vi "ChemProj.vi"() -> ()   [LabVIEW 2012]
uses:
  <userlib>/ImageProcessing/InitCamera_NTSC.vi
  <userlib>/ImageProcessing/FilterGreenPlane.vi
  <userlib>/ImageProcessing/FilterRedPlane.vi
panel:
  out "Question":string
  out "Element Found":string[](array[string])
  out "Grade":dbl
  out "Element":string[](array[string])
  out "indexsWhereTrue":i32[](array[numeric])
  out "Min":dbl[](array[numeric])
  out "Max":dbl[](array[numeric])
  out "x+y":dbl[](array[numeric])
  out "S4":dbl[](array[numeric])
  out "S3":dbl[](array[numeric])
  out "S2":dbl[](array[numeric])
  out "S1":dbl[](array[numeric])
  in  "Path":path
  out "Periodic":string[][](array[string])
  out "image 2":picture
  out "Ra4":dbl
  out "Ra3":dbl
  out "Ra2":dbl
  out "Ra1":dbl
  out "A4":dbl
  out "A3":dbl
  out "A2":dbl
  out "A1":dbl
  out "a4":dbl
  out "a3":dbl
  out "a2":dbl
  out "a1":dbl
  out "Centroid 4":cluster{"X":dbl, "Y":dbl}
  out "Centroid 3":cluster{"X":dbl, "Y":dbl}
  out "Centroid 2":cluster{"X":dbl, "Y":dbl}
  out "Centroid":cluster{"X":dbl, "Y":dbl}
  out "initialized array 2":dbl[][](array[numeric])
  out "image":picture
  in  "Stop":bool
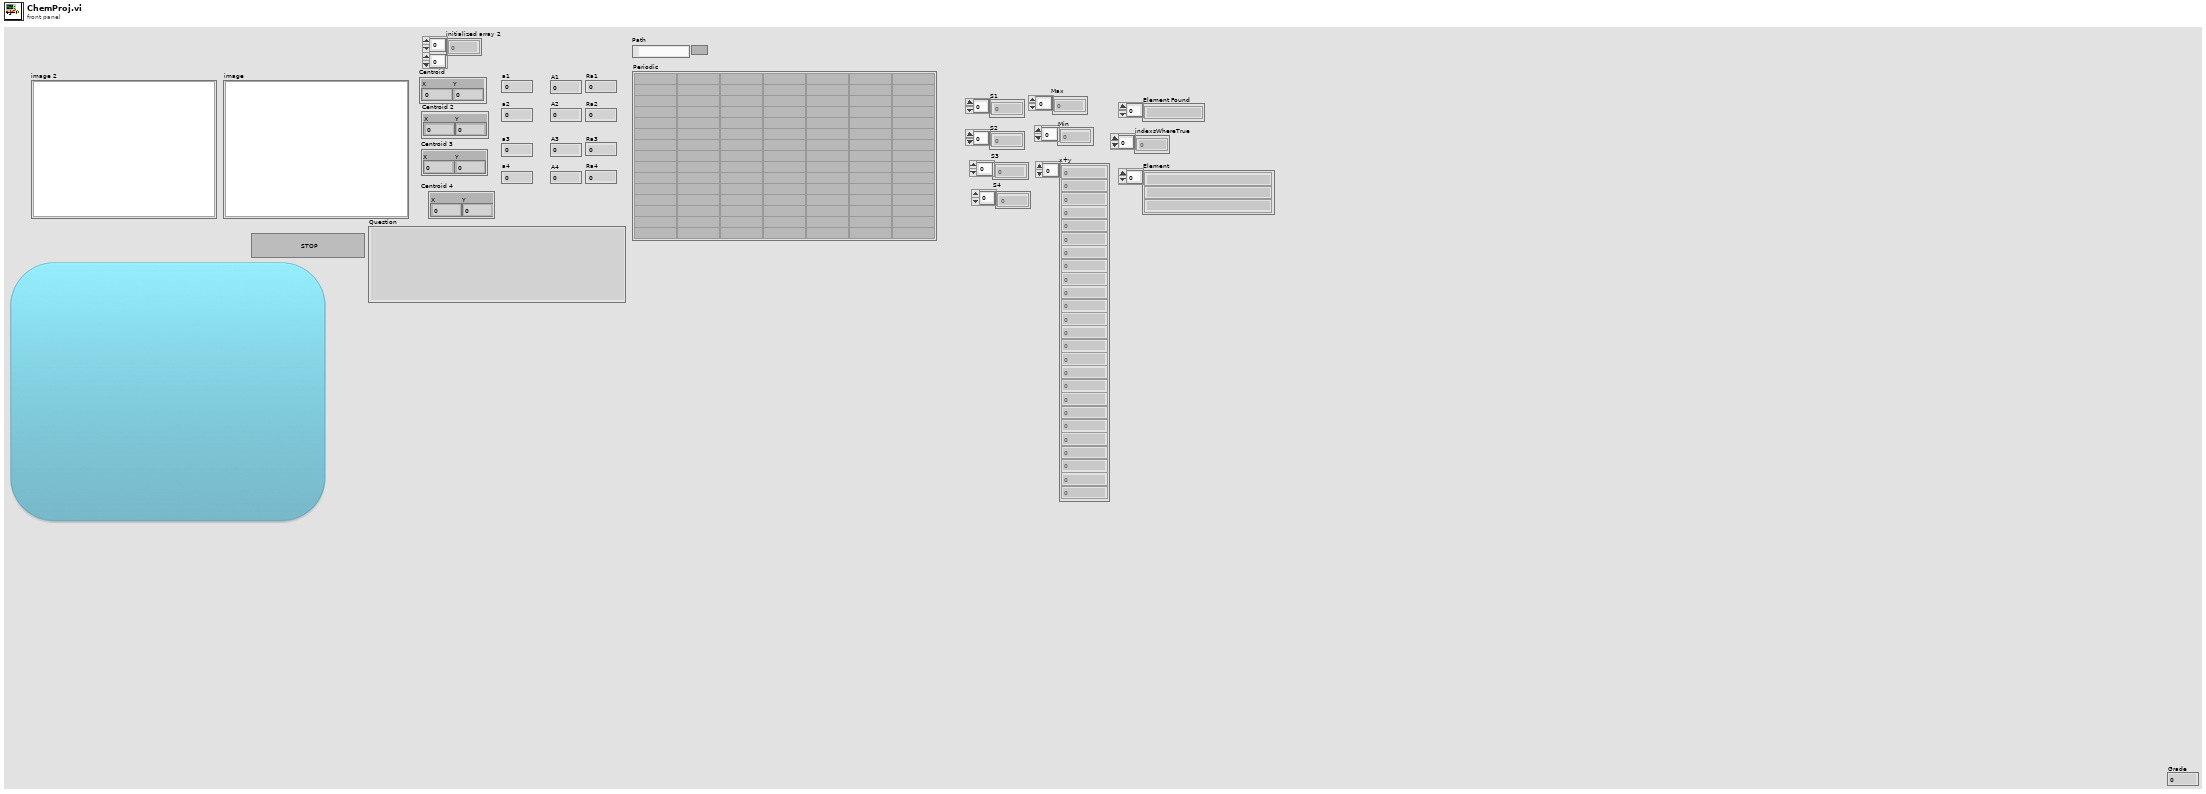
[diagram p1: front panel]
types:
  T1 = typedef "QT_Ref.ctl" = refnum<k1>
  T2 = cluster{"Width":u16, "Style":enum32{"Solid", "Dash", "Dot", "DashDot", "DashDotDot"}}
  T3 = typedef "QT_Image.ctl" = cluster{"Width":i32, "Height":i32, "Depth":i32, "data":u8[], "Compressed data":u8[], "Color table":u32[], "Duration":i32, "Options":i32, "Timestamp":i32, "ID":i32, "Reserved":i32, "Dialogs":u32}
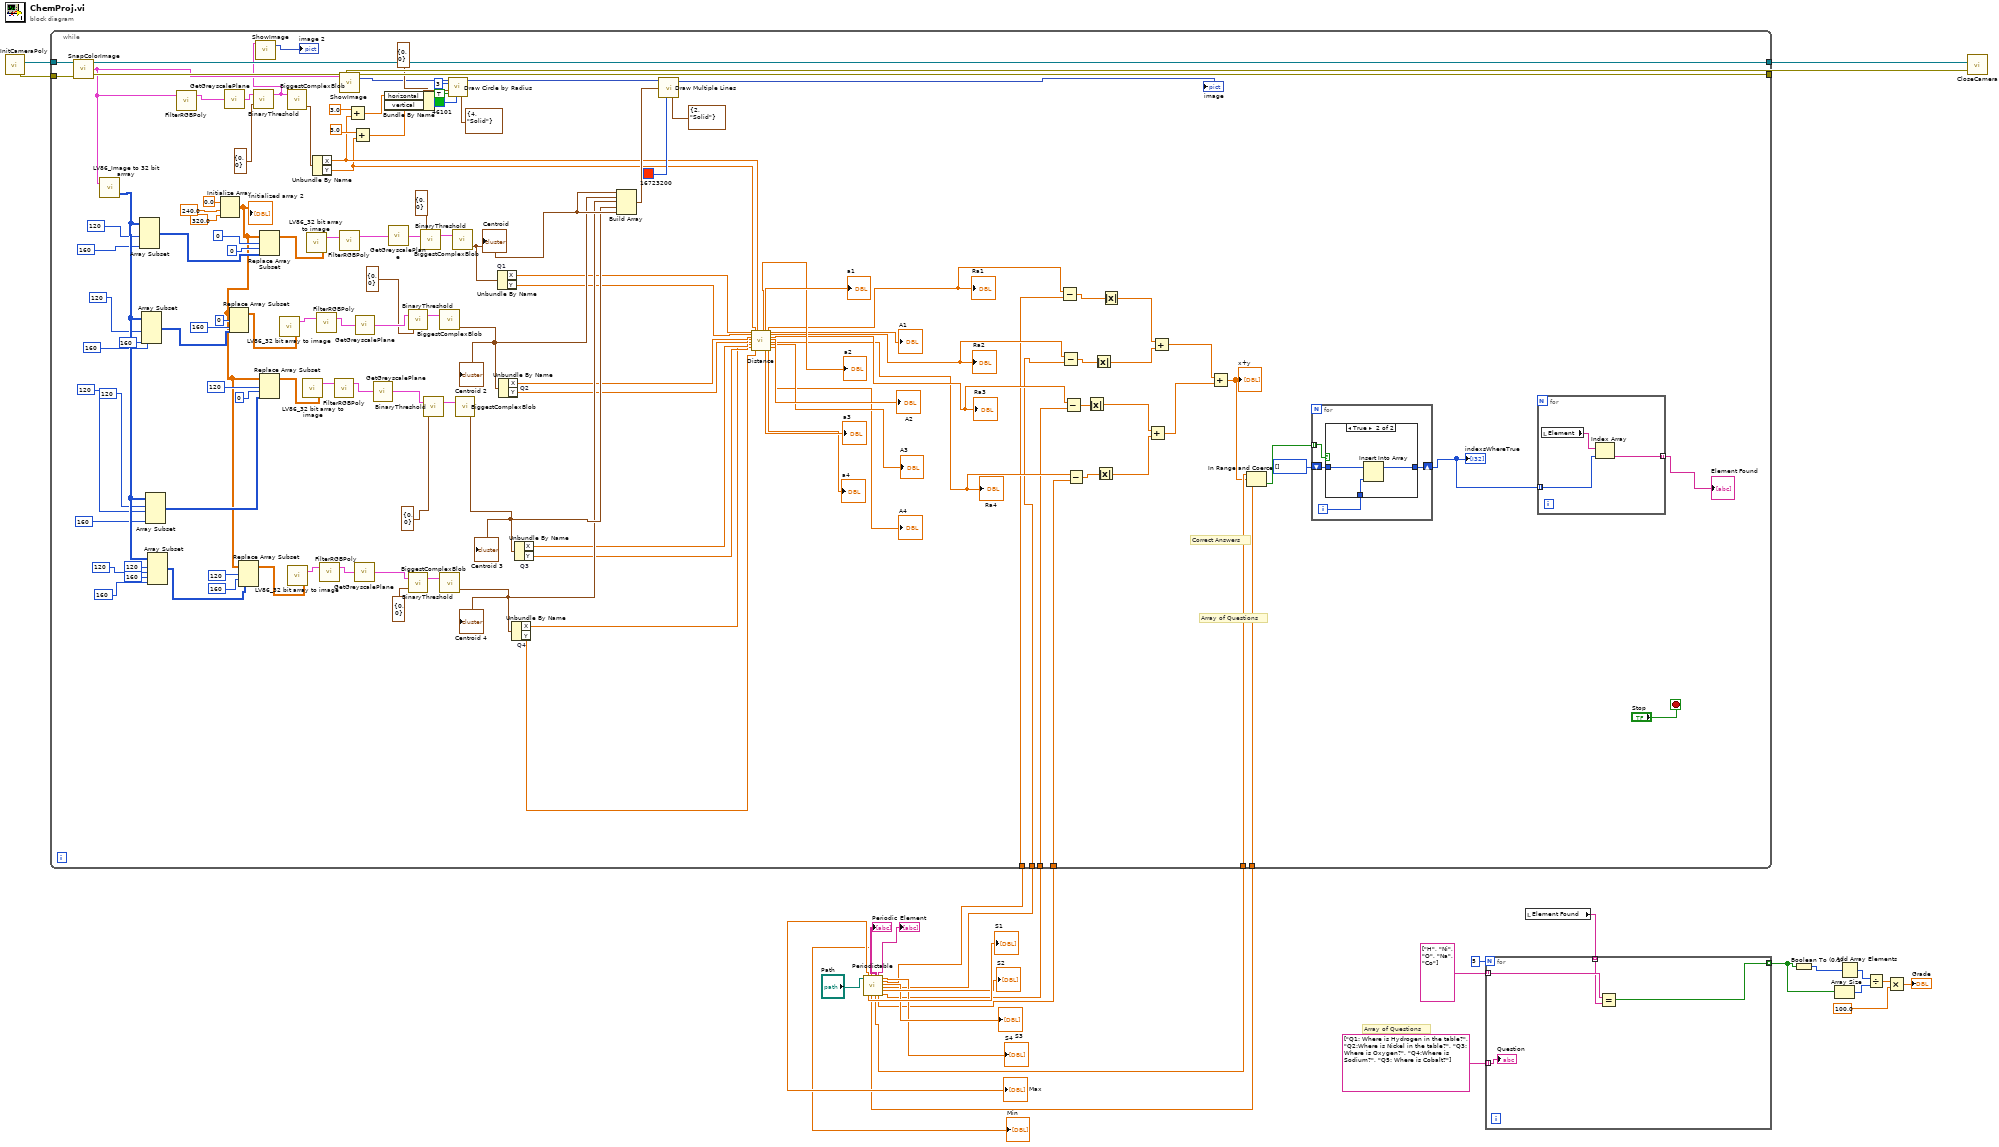
[diagram p0: block diagram]
diagram:
  # "Array of Questions"
  n1 = call-poly <userlib>:"InitCameraPoly.vi"() -> ("error out"=w27:errorcluster, "QT Ref Out"=w28:T1)  [unwired: 2 in]
  n2 = call "Periodictable.vi"("Path"="Path") -> ("Max"=→"Max":dbl[], "S1"=→"S1":dbl[], "Min"=→"Min":dbl[], "Array"=w17:dbl[], "Periodic"=→"Periodic":string[][], "Array 2"=w16:dbl[], "Element"=→"Element":string[], "Array 3"=w12:dbl[], "S4"=→"S4":dbl[], "Array 6"=w15:dbl[], "S3"=→"S3":dbl[], "Array 5"=w14:dbl[], "S2"=→"S2":dbl[], "Array 4"=w13:dbl[])  [unwired: 5 in]
  n3 = while {
    tunnel: w27 -> [w158]
    tunnel: w28 -> [w157]
    tunnel: [w156] -> w29
    tunnel: [w155] -> w30
    tunnel: w15 -> [w51]
    tunnel: w14 -> [w50]
    tunnel: w13 -> [w49]
    tunnel: w12 -> [w48]
    tunnel: w16 -> [w37]
    tunnel: w17 -> [w36]
    stop <- "Stop" stop-if-true
    # "Correct Answers"
    # "Array of Questions"
    n4 = call <userlib>:"SnapColorImage.vi"("error in (no error)"=w158, "QT Ref In"=w157) -> ("error out"=w156:errorcluster, "Image Out"=w89:T3, "QT Ref Out"=w155:T1)  [unwired: 1 in]
    n5 = call <userlib>:"LV86_Image to 32 bit arrray.vi"("Image In"=w89) -> ("Intensity Graph"=w153:u32[][])  [unwired: 1 in, 1 out]
    n6 = Array Subset(array=w153, length (row)=120 ("length"), length (col)=160 ("length")) -> (w129:u32[][])  [unwired: 2 in]
    n7 = Array Subset(array=w153, length (row)=120 ("length"), index (col)=160 ("index"), length (col)=160 ("length")) -> (w140:u32[][])  [unwired: 1 in]
    n8 = Array Subset(array=w153, index (row)=120 ("index"), length (row)=120 ("length"), length (col)=160 ("length")) -> (w123:u32[][])  [unwired: 1 in]
    n9 = Array Subset(array=w153, index (row)=120 ("index"), length (row)=120 ("length"), index (col)=160 ("index"), length (col)=160 ("length")) -> (w120:u32[][])
    n10 = call-poly <userlib>:"FilterRGBPoly.vi"("Image in"=w89) -> ("Image out"=w92:T3)  [unwired: 1 in, 1 out]
    n11 = Initialize Array(0.0 ("element"), 240.0 ("element"), 320.0 ("element")) -> (w119:dbl[][])
    "initialized array 2" <- w119
    n12 = call <userlib>:"GetGreyscalePlane.vi"("Image In"=w92) -> ("Greyscale  Out"=w76:T3)
    n13 = Replace Array Subset(array=w119, new element=w140, index (row)=0, index (col)=160 ("index (row)")) -> (w139:dbl[][])
    n14 = Replace Array Subset(array=w119, new element=w120, index (row)=120, index (col)=160 ("index (row)")) -> (w117:dbl[][])
    n15 = call <userlib>:"BinaryThreshold.vi"("threshold"=cluster{u8, u8} {0, 0}, "Image In"=w76) -> ("Image Out"=w74:T3)  [unwired: 1 in]
    n16 = call <userlib>:"ShowImage.vi"("Image"=w74) -> ("image"=→"image 2":picture)  [unwired: 2 in, 1 out]
    n17 = Replace Array Subset(array=w119, new element=w129, index (row)=0, index (col)=0 ("index (row)")) -> (w128:dbl[][])
    n18 = Replace Array Subset(array=w119, new element=w123, index (row)=120, index (col)=0 ("index (row)")) -> (w118:dbl[][])
    n19 = call <userlib>:"LV86_32 bit array to image.vi"("Intensity Graph"=w139) -> ("Image Out"=w116:T3)  [unwired: 2 in]
    n20 = call <userlib>:"BiggestComplexBlob.vi"("Image in"=w74) -> ("Centroid"=w90:cluster{"X":dbl, "Y":dbl})  [unwired: 1 in, 2 out]
    n21 = call <userlib>:"LV86_32 bit array to image.vi"("Intensity Graph"=w117) -> ("Image Out"=w114:T3)  [unwired: 2 in]
    n22 = call <userlib>:"LV86_32 bit array to image.vi"("Intensity Graph"=w118) -> ("Image Out"=w115:T3)  [unwired: 2 in]
    n23 = call <userlib>:"LV86_32 bit array to image.vi"("Intensity Graph"=w128) -> ("Image Out"=w127:T3)  [unwired: 2 in]
    n24 = Unbundle By Name(w90) -> ("X"=w73:dbl, "Y"=w72:dbl)
    n25 = call-poly <userlib>:"FilterRGBPoly.vi"("Image in"=w116) -> ("Image out"=w113:T3)  [unwired: 1 in, 1 out]
    n26 = call-poly <userlib>:"FilterRGBPoly.vi"("Image in"=w114) -> ("Image out"=w111:T3)  [unwired: 1 in, 1 out]
    n27 = call-poly <userlib>:"FilterRGBPoly.vi"("Image in"=w115) -> ("Image out"=w112:T3)  [unwired: 1 in, 1 out]
    n28 = call <userlib>:"ShowImage.vi"("Image"=w89) -> ("image"=w77:picture)  [unwired: 2 in, 1 out]
    n29 = call-poly <userlib>:"FilterRGBPoly.vi"("Image in"=w127) -> ("Image out"=w126:T3)  [unwired: 1 in, 1 out]
    n30 = Add(x=3.0, y=w73) -> (x+y=w83:dbl)
    n31 = Add(x=3.0, y=w72) -> (x+y=w82:dbl)
    n32 = call <userlib>:"GetGreyscalePlane.vi"("Image In"=w111) -> ("Greyscale  Out"=w105:T3)
    n33 = call <userlib>:"GetGreyscalePlane.vi"("Image In"=w113) -> ("Greyscale  Out"=w107:T3)
    n34 = call <userlib>:"GetGreyscalePlane.vi"("Image In"=w112) -> ("Greyscale  Out"=w106:T3)
    n35 = Bundle By Name(cluster=cluster{"horizontal":i16, "vertical":i16} {"horizontal"=0, "vertical"=0} ("pixel center"), "horizontal"=w83, "vertical"=w82) -> (w87:cluster{"horizontal":i16, "vertical":i16})
    n36 = call <userlib>:"GetGreyscalePlane.vi"("Image In"=w126) -> ("Greyscale  Out"=w125:T3)
    n37 = call <userlib>:"BinaryThreshold.vi"("threshold"=cluster{u8, u8} {0, 0}, "Image In"=w107) -> ("Image Out"=w110:T3)  [unwired: 1 in]
    n38 = call <userlib>:"BinaryThreshold.vi"("threshold"=cluster{u8, u8} {0, 0}, "Image In"=w105) -> ("Image Out"=w108:T3)  [unwired: 1 in]
    n39 = call <userlib>:"BinaryThreshold.vi"("threshold"=cluster{u8, u8} {0, 0}, "Image In"=w125) -> ("Image Out"=w124:T3)  [unwired: 1 in]
    n40 = call <userlib>:"BinaryThreshold.vi"("threshold"=cluster{u8, u8} {0, 0}, "Image In"=w106) -> ("Image Out"=w109:T3)  [unwired: 1 in]
    n41 = call <userlib>:"BiggestComplexBlob.vi"("Image in"=w110) -> ("Centroid"=w95:cluster{"X":dbl, "Y":dbl})  [unwired: 1 in, 2 out]
    "Centroid 2" <- w95
    n42 = call <userlib>:"BiggestComplexBlob.vi"("Image in"=w108) -> ("Centroid"=w93:cluster{"X":dbl, "Y":dbl})  [unwired: 1 in, 2 out]
    "Centroid 4" <- w93
    n43 = call <vilib>:"Draw Circle by Radius.vi"("pen"=T2 {"Width"=4, "Style"=enum."Solid"}, "color(black)"=u32 46101, "fill?(F)"=TRUE, "pixel center"=w87, "radius"=i16 3, "picture"=w77) -> ("new picture"=w88:picture)  [unwired: 5 in]
    n44 = call <userlib>:"BiggestComplexBlob.vi"("Image in"=w124) -> ("Centroid"=w96:cluster{"X":dbl, "Y":dbl})  [unwired: 1 in, 2 out]
    "Centroid" <- w96
    n45 = call <userlib>:"BiggestComplexBlob.vi"("Image in"=w109) -> ("Centroid"=w94:cluster{"X":dbl, "Y":dbl})  [unwired: 1 in, 2 out]
    "Centroid 3" <- w94
    n46 = Unbundle By Name "Q1"(w96) -> ("X"=w71:dbl, "Y"=w70:dbl)
    n47 = Unbundle By Name "Q2"(w95) -> ("X"=w69:dbl, "Y"=w68:dbl)
    n48 = Unbundle By Name "Q4"(w93) -> ("X"=w65:dbl, "Y"=w64:dbl)
    n49 = Unbundle By Name "Q3"(w94) -> ("X"=w67:dbl, "Y"=w66:dbl)
    n50 = Build Array(w96, w95, w93, w94, w96) -> (w103:cluster{"X":dbl, "Y":dbl}[])
    n51 = call <vilib>:"Draw Multiple Lines.vi"("picture"=w88, "line endpoints"=w103, "color(black)"=u32 16723200, "pen"=T2 {"Width"=2, "Style"=enum."Solid"}) -> ("new picture"=→"image":picture)  [unwired: 5 in]
    n52 = call "Distance.vi"("X1"=w71, "Y1"=w70, "X2"=w69, "Y2"=w68, "X3"=w67, "Y3"=w66, "x4"=w65, "Y"=w72, "Y4"=w64, "X"=w73) -> ("a2"=→"a2":dbl, "a1"=→"a1":dbl, "a3"=→"a3":dbl, "Ra1"=w55:dbl, "a4"=→"a4":dbl, "A1"=→"A1":dbl, "Ra2"=w54:dbl, "Ra3"=w53:dbl, "A2"=→"A2":dbl, "Ra4"=w52:dbl, "A3"=→"A3":dbl, "A4"=→"A4":dbl)  [unwired: 6 in]
    "Ra1" <- w55
    "Ra2" <- w54
    "Ra3" <- w53
    "Ra4" <- w52
    n53 = Subtract(x=w55, y=w51) -> (x-y=w47:dbl[])
    n54 = Subtract(x=w54, y=w50) -> (x-y=w46:dbl[])
    n55 = Subtract(x=w53, y=w49) -> (x-y=w45:dbl[])
    n56 = Subtract(x=w52, y=w48) -> (x-y=w44:dbl[])
    n57 = Absolute Value(x=w45) -> (abs(x)=w41:dbl[])
    n58 = Absolute Value(x=w46) -> (abs(x)=w42:dbl[])
    n59 = Absolute Value(x=w44) -> (abs(x)=w40:dbl[])
    n60 = Absolute Value(x=w47) -> (abs(x)=w43:dbl[])
    n61 = Add(x=w41, y=w40) -> (x+y=w38:dbl[])
    n62 = Add(x=w43, y=w42) -> (x+y=w39:dbl[])
    n63 = Add(x=w39, y=w38) -> (x+y=w35:dbl[])
    "x+y" <- w35
    n64 = In Range and Coerce(upper limit=w37, x=w35, lower limit=w36) -> (In Range?=w33:bool[])  [unwired: 1 out]
    n65 = for {
      shift-right: [w164] -> w34
      shift-left: i32[] [] -> [w163]
      tunnel: w33 -> [w162] mode=indexing
      i -> [w165]
      n66 = case shown="True" w162 {
        tunnel: w165 -> [_ w169]
        tunnel: [w166 w168] -> w164
        tunnel: w163 -> [w166 w167]
        frame False {
        }
        frame True {
          n67 = Insert Into Array(array=w167, new element=w169) -> (w168:i32[])  [unwired: 1 in]
        }
      }
    }
    "indexsWhereTrue" <- w34
    n68 = for {
      tunnel: w34 -> [w161] mode=indexing
      tunnel: [w159] -> w31 mode=indexing
      n69 = local read "Element"() -> (w160:string[])
      n70 = Index Array(array=w160, index=w161) -> (element=w159:string)
    }
    "Element Found" <- w31
  }
  n71 = local read "Element Found"() -> (w2:string[])
  n72 = for {
    N: 5 -> [_]
    tunnel: [w173] -> w10 mode=indexing
    tunnel: string[] ["H", "Ni", "O", "Na", "Co"] -> [w172] mode=indexing
    tunnel: w2 -> [w171] mode=indexing
    tunnel: string[] ["Q1: Where is Hydrogen in the table?", "Q2:Where is Nickel in the table?", "Q3: Where is Oxygen?", "Q4:Where is Sodium?", "Q5: Where is Cobalt?"] -> [w170] mode=indexing
    n73 = Equal?(x=w172, y=w171) -> (x = y?=w173:bool)
    "Question" <- w170
  }
  n74 = Boolean To (0,1)(Boolean=w10) -> (0, 1=w9:i16[])
  n75 = Array Size(array=w10) -> (size(s)=w5:i32)
  n76 = Add Array Elements(numeric array=w9) -> (sum=w4:i16)
  n77 = Divide(x=w4, y=w5) -> (x/y=w6:dbl)
  n78 = Multiply(x=w6, y=100.0) -> (x*y=→"Grade":dbl)
  n79 = call <userlib>:"CloseCamera.vi"("error in (no error)"=w29, "QT Ref In"=w30) -> ()  [unwired: 1 in, 1 out]
